vi "LoadAutoRoutine.vi"(10 "RoutineName":string) -> (2 "Array":T1[](array[typedef]))   [LabVIEW 2023]
uses:
  Support Code/Auto_Action.ctl
  <vilib>/Utility/config.llb/Read Key (String).vi
  <vilib>/Utility/config.llb/Read Key (Double).vi
  <vilib>/Utility/config.llb/NI_LVConfig.lvlib
panel:
  out "Numeric":i32
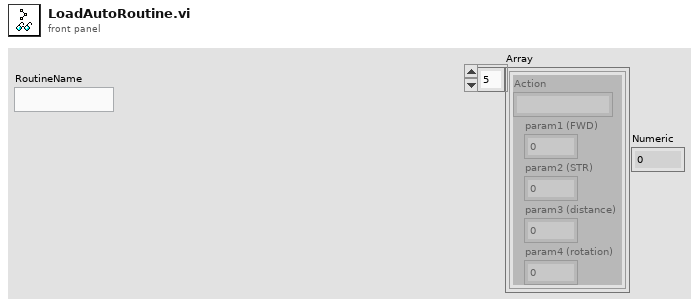
[diagram p1: front panel]
types:
  T1 = typedef "Auto_Action.ctl" = cluster{"Action":string, "param1 (FWD)":dbl, "param2 (STR)":dbl, "param3 (distance)":dbl, "param4 (rotation)":dbl}
  T2 = typedef "NI_LVConfig.lvlib/Config Data RefNum.ctl" = refnum<k1>
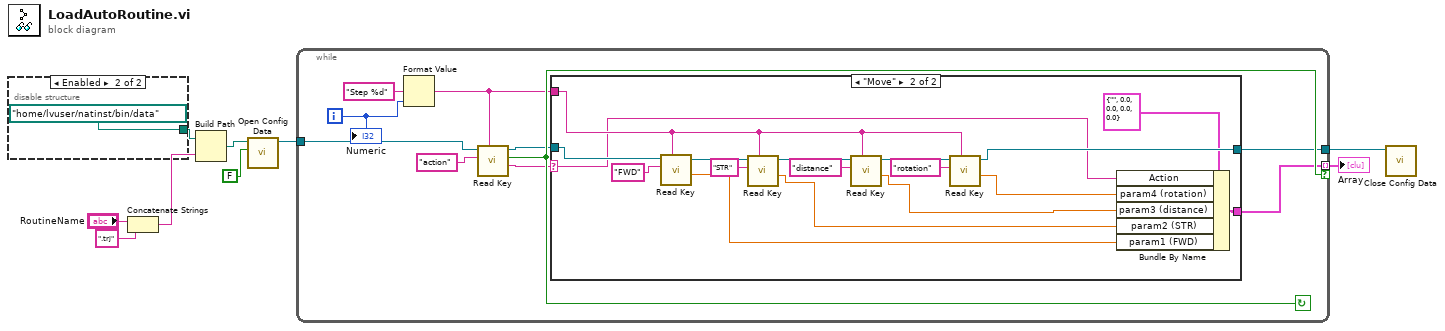
[diagram p0: block diagram]
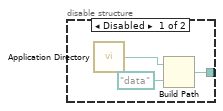
[diagram p2: hidden frame]
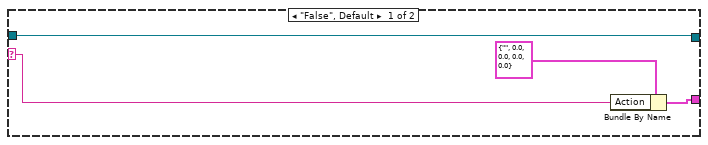
[diagram p3: hidden frame]
diagram:
  n1 = disable-structure shown="Enabled" {
    disable-tunnel: [w10 path "/home/lvuser/natinst/bin/data" ("appended path")] -> w9
    frame Disabled {
      n2 = call <vilib>:"Application Directory.vi"() -> ("Application Directory"=w12:path)
      n3 = Build Path(base path=w12, name or relative path=path "data") -> (appended path=w10:path)
    }
    frame Enabled {
    }
  }
  n4 = Concatenate Strings("RoutineName", ".trj" ("string")) -> (w3:string)
  n5 = Build Path(base path=w9, name or relative path=w3) -> (appended path=w8:path)
  n6 = call <vilib>:"Open Config Data.vi"("create file if necessary (T)"=FALSE, "configuration file path"=w8) -> ("refnum"=w6:T2)  [unwired: 7 in, 2 out]
  n7 = while {
    tunnel: w6 -> [w21]
    tunnel: [w15] -> w5
    tunnel: [w14] -> w4 mode=indexing if=w19
    i -> [w20]
    stop <- w19 continue-if-true
    n8 = Format Value(format string="Step %d", value (0)=w20) -> (output string=w16:string)  [unwired: 1 in]
    n9 = call-poly <vilib>:"Read Key.vi"("section"=w16, "key"="action", "refnum"=w21) -> ("value"=w18:string, "found?"=w19:bool, "refnum out"=w17:T2)  [unwired: 5 in, 1 out]
    n10 = case shown="\"Move\"" w18 {
      selector: w18 -> [w24 w34]
      tunnel: w17 -> [w27 w37]
      tunnel: w16 -> [_ w36]
      tunnel: [w27 w35] -> w15
      tunnel: [w25 w28] -> w14
      frame "False", Default {
        n11 = Bundle By Name(cluster=T1 {"Action"="", "param1 (FWD)"=0.0, "param2 (STR)"=0.0, "param3 (distance)"=0.0, "param4 (rotation)"=0.0} ("output cluster"), "Action"=w24) -> (w25:T1)
      }
      frame "Move" {
        n12 = call-poly <vilib>:"Read Key.vi"("section"=w36, "key"="FWD", "refnum"=w37) -> ("value"=w29:dbl, "refnum out"=w43:T2)  [unwired: 5 in, 2 out]
        n13 = call-poly <vilib>:"Read Key.vi"("section"=w36, "key"="STR", "refnum"=w43) -> ("value"=w31:dbl, "refnum out"=w44:T2)  [unwired: 5 in, 2 out]
        n14 = call-poly <vilib>:"Read Key.vi"("section"=w36, "key"="distance", "refnum"=w44) -> ("value"=w30:dbl, "refnum out"=w42:T2)  [unwired: 5 in, 2 out]
        n15 = call-poly <vilib>:"Read Key.vi"("section"=w36, "key"="rotation", "refnum"=w42) -> ("value"=w32:dbl, "refnum out"=w35:T2)  [unwired: 5 in, 2 out]
        n16 = Bundle By Name(cluster=T1 {"Action"="", "param1 (FWD)"=0.0, "param2 (STR)"=0.0, "param3 (distance)"=0.0, "param4 (rotation)"=0.0} ("output cluster"), "Action"=w34, "param4 (rotation)"=w32, "param3 (distance)"=w30, "param2 (STR)"=w31, "param1 (FWD)"=w29) -> (w28:T1)
      }
    }
    "Numeric" <- w20
  }
  "Array" <- w4
  n17 = call <vilib>:"Close Config Data.vi"("refnum"=w5) -> ()  [unwired: 9 in, 2 out]
